vi "Resolve Pin Map Path.vi"(8 "error in":errorcluster, 10 "Pin Map Path":string, 11 "Sequence Context In":refnum<k7>) -> (0 "error out":errorcluster, 3 "Pin Map Path":string)   [LabVIEW 2020, in "NIDigitalBurstPattern.lvlib"]
uses:
  NIDigitalBurstPattern.lvlib
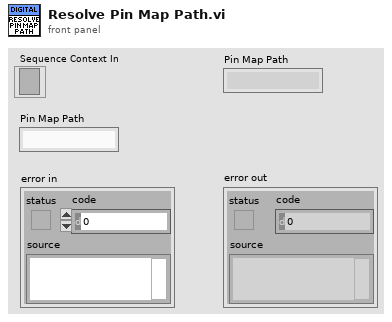
[diagram p1: front panel]
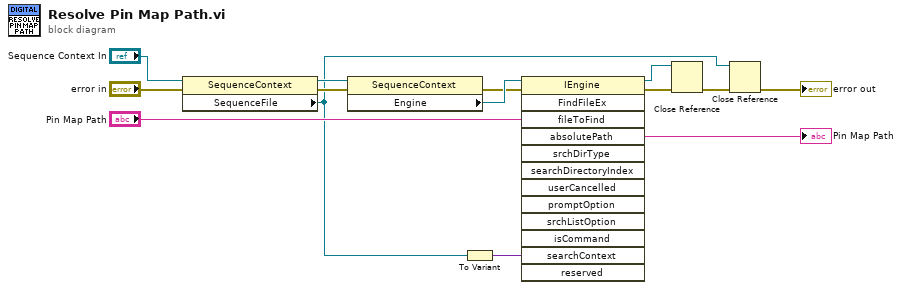
[diagram p0: block diagram]
diagram:
  n1 = property class="SequenceContext"(reference="Sequence Context In", error in="error in") -> (reference out=w5:refnum<k7>, error out=w7:errorcluster, "SequenceFile"=w2:refnum<k7>)
  n2 = property class="SequenceContext"(reference=w5, error in=w7) -> (error out=w12:errorcluster, "Engine"=w13:refnum<k7>)  [unwired: 1 out]
  n3 = To Variant(anything=w2) -> (Variant=w1:variant)
  n4 = invoke class="IEngine" method="FindFileEx"(reference=w13, error in=w12, "fileToFind"="Pin Map Path", "searchContext"=w1) -> (reference out=w10:refnum<k7>, error out=w9:errorcluster, "absolutePath"=→"Pin Map Path":string)  [unwired: 9 in, 10 out]
  n5 = Close Reference(reference=w10, error in (no error)=w9) -> (error out=w4:errorcluster)
  n6 = Close Reference(reference=w2, error in (no error)=w4) -> (error out=→"error out":errorcluster)
